vi "TestPCO.Cam.vi"() -> ()   [LabVIEW 2011]
uses:
  <vilib>/Utility/importsl/GetValueByPointer/datatype.ctl
  <vilib>/Utility/importsl/GetValueByPointer/GetValueByPointer.xnode
  National Instruments/LabVIEW 2011/resource/lvimptsl.dll
panel:
  out "End":bool
  in  "Exposure [ms]":dbl(slide) scale=1.0..100.0
  out "ActRes":cluster{"wXResAct":u16, "wYResAct":u16}
  out "Exposure [s]":dbl
  out "ImgPointer":u32
  out "sBufNr out":i16
  in  "Finish":bool
  out "Intensity Graph":u16[][](graph)
  out "bytes allocated":u32
  out "Frame":i32
  out "Handle":u64
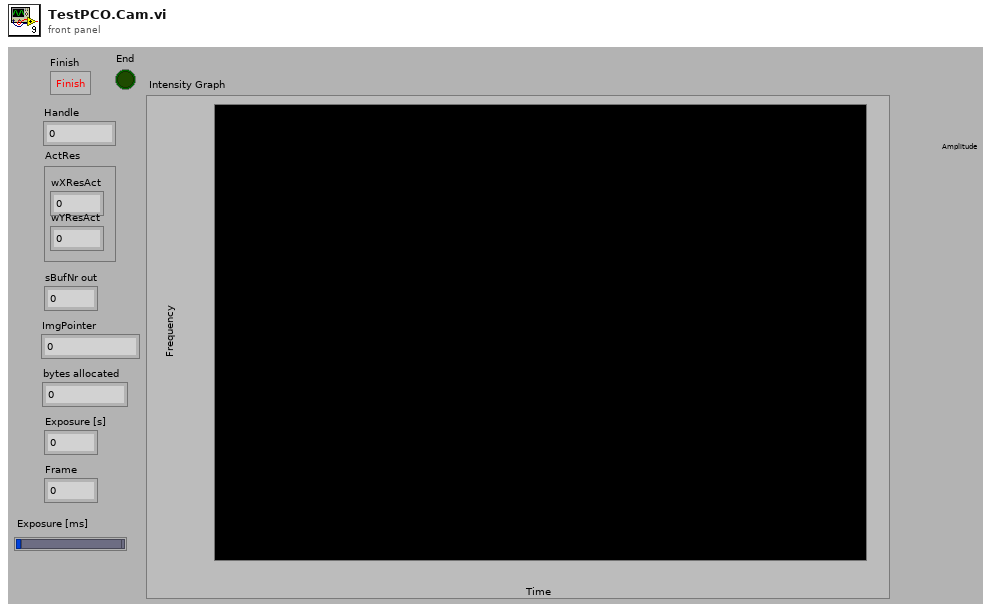
[diagram p1: front panel]
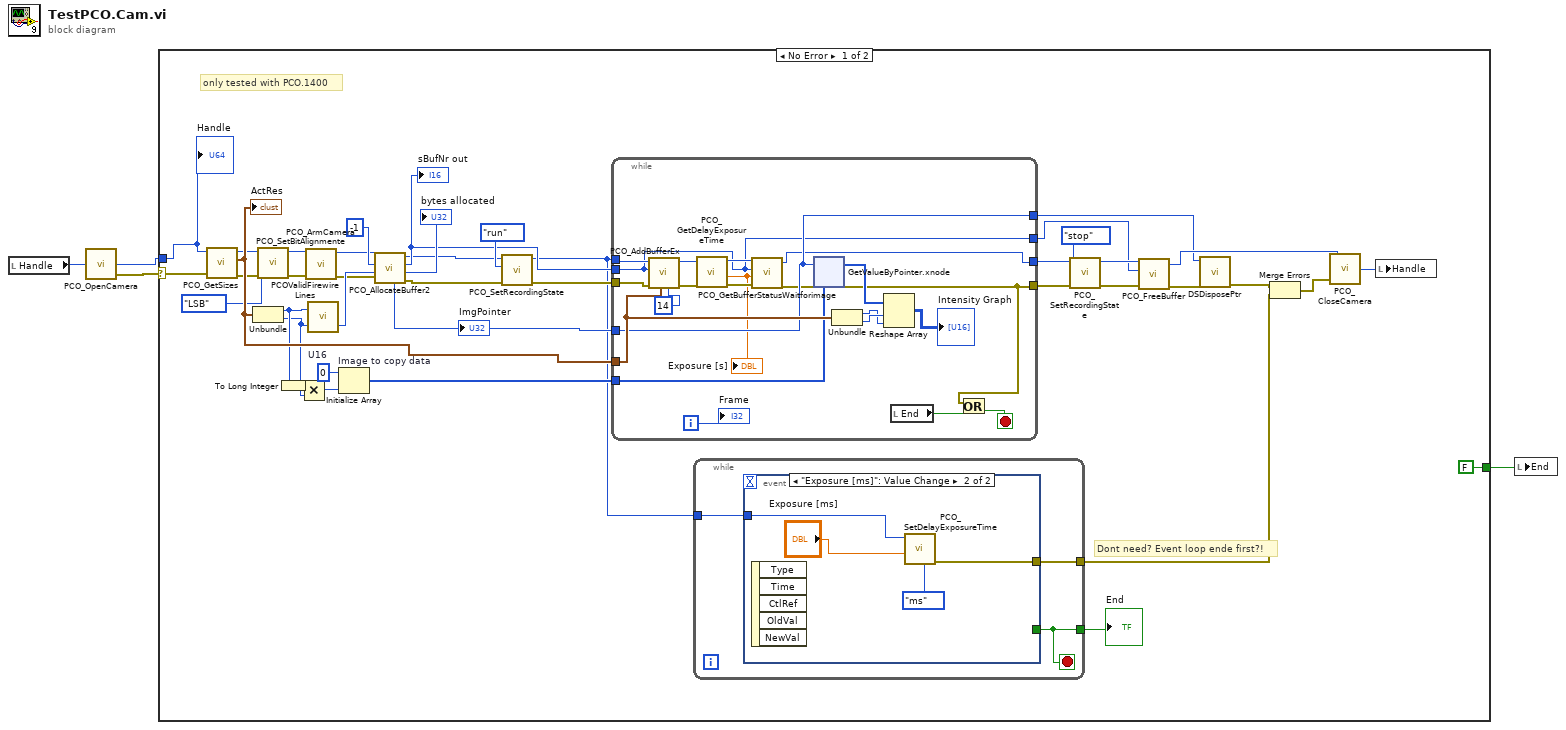
[diagram p0: block diagram]
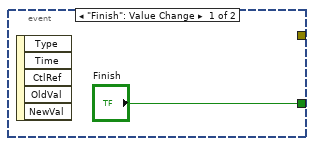
[diagram p2: hidden frame]
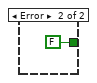
[diagram p3: hidden frame]
diagram:
  n1 = local read "Handle"() -> (w2:u64)
  n2 = call "PCO_OpenCamera.vi"("Handle (0 for new)"=w2) -> ("error out"=w4:errorcluster, "Handle Out"=w3:u64)  [unwired: 2 in, 1 out]
  n3 = case shown="No Error" w4 {
    selector: w4 -> [w34 _]
    tunnel: w3 -> [w33 _]
    tunnel: [FALSE ("End") FALSE ("End")] -> w1
    frame No Error {
      w27 = u16 0  # U16
      # "Dont need? Event loop ende first?!"
      # "only tested with PCO.1400"
      n4 = call "PCO_GetSizes.vi"("error in (no error)"=w34, "Handle"=w33) -> ("error out"=w7:errorcluster, "ActRes"=w32:cluster{"wXResAct":u16, "wYResAct":u16}, "Handle Out"=w9:u64)  [unwired: 7 out]
      "ActRes" <- w32
      n5 = Unbundle(w32) -> ("wXResAct"=w30:u16, "wYResAct"=w29:u16)
      n6 = call "PCO_SetBitAlignmente.vi"("error in (no error)"=w7, "wBitAlignment"=enum16{"MSB", "LSB"}."LSB", "Handle"=w9) -> ("error out"=w6:errorcluster, "Handle Out"=w8:u64)  [unwired: 6 in, 1 out]
      n7 = To Long Integer(number=w30) -> (32bit integer=w17:i32)
      n8 = Multiply(x=w17, y=w29) -> (x*y=w28:i32)
      n9 = call "PCO_ArmCamera.vi"("error in (no error)"=w6, "Handle"=w8) -> ("error out"=w21:errorcluster, "Handle Out"=w22:u64)  [unwired: 8 out]
      n10 = call "PCOValidFirewireLines.vi"("wYResAct"=w29, "wXResAct"=w30) -> ("ValidBytes"=w31:u32)  [unwired: 1 out]
      n11 = Initialize Array "Image to copy data"(w27, w28) -> (w26:u16[])
      n12 = call "PCO_AllocateBuffer2.vi"("error in (no error)"=w21, "PointerSize (bytes)"=w31, "sBufNr"=i16 -1, "Handle"=w22) -> ("error out"=w20:errorcluster, "bytes allocated"=→"bytes allocated":u32, "sBufNr out"=w35:i16, "Handle Out"=w19:u64, "BufferPointer"=w43:u64)  [unwired: 3 out]
      "sBufNr out" <- w35
      "ImgPointer" <- w43
      n13 = call "PCO_SetRecordingState.vi"("error in (no error)"=w20, "wRecState"=enum16{"stop", "run"}."run", "Handle"=w19) -> ("error out"=w38:errorcluster, "Handle Out"=w13:u64)  [unwired: 7 out]
      n14 = while {
        tunnel: w13 -> [w69]
        tunnel: [w60] -> w42
        tunnel: [w55] -> w41
        tunnel: w43 -> [w66]
        tunnel: w35 -> [w58]
        tunnel: w32 -> [w68]
        tunnel: w38 -> [w71]
        tunnel: w26 -> [w67]
        tunnel: [w66] -> w23
        tunnel: [w58] -> w18
        i -> [w75]
        stop <- w56 stop-if-true
        n15 = call "PCO_AddBufferEx.vi"("BitPerPixel"=u16 14, "Resolution"=w68, "error in (no error)"=w71, "sBufNr"=w58, "Handle"=w69) -> ("error out"=w64:errorcluster, "Handle Out"=w65:u64)  [unwired: 1 in, 4 out]
        n16 = call "PCO_GetDelayExposureTime.vi"("error in (no error)"=w64, "Handle"=w65) -> ("error out"=w63:errorcluster, "Exposure [s]"=w61:dbl, "Handle Out"=w62:u64)  [unwired: 7 out]
        "Exposure [s]" <- w61
        n17 = call "PCO_GetBufferStatusWaitforimage.vi"("error in"=w63, "expected seconds"=w61, "sBufNr"=w58, "Handle"=w62) -> ("error out"=w59:errorcluster, "Handle Out"=w60:u64)  [unwired: 1 out]
        n18 = xnode "GetValueByPointer.xnode"("Pointer"=w66, "InputType"=w67, "ErrorIn"=w59) -> ("Output"=w57:u16[], "ErrorOut"=w55:errorcluster)  [unwired: 1 in]
        n19 = Unbundle(w68) -> ("wXResAct"=w73:u16, "wYResAct"=w74:u16)
        n20 = Reshape Array(w57, w74, w73) -> (→"Intensity Graph":u16[][])
        n21 = local read "End"() -> (w54:bool)
        n22 = Or(x=w55, y=w54) -> (x .or. y?=w56:bool)
        "Frame" <- w75
      }
      n23 = while {
        tunnel: [w48] -> w15
        tunnel: w13 -> [w47]
        tunnel: [w46] -> w10
        stop <- w48 stop-if-true
        n24 = event shown="[1] \"Exposure [ms]\": Value Change" {
          selector: _ -> [_ _]
          dyn-events: _ -> [_ _]
          timeout: _ -> [_ _]
          tunnel: ["Finish" _] -> w48
          tunnel: w47 -> [_ w53]
          tunnel: [_ w50] -> w46
          event "Finish": Value Change {
            n25 = event-data() -> ()  [unwired: 1 in, 5 out]
          }
          event "Exposure [ms]": Value Change {
            n26 = event-data() -> ()  [unwired: 1 in, 5 out]
            n27 = call "PCO_SetDelayExposureTime.vi"("wTimebaseExposure"=enum16{"ns", "µs", "ms"}."ms", "dwExposure"="Exposure [ms]", "Handle"=w53) -> ("error out"=w50:errorcluster)  [unwired: 6 in, 2 out]
          }
        }
      }
      "End" <- w15
      n28 = call "PCO_SetRecordingState.vi"("error in (no error)"=w41, "wRecState"=enum16{"stop", "run"}."stop", "Handle"=w42) -> ("error out"=w37:errorcluster, "Handle Out"=w36:u64)  [unwired: 7 out]
      n29 = call "PCO_FreeBuffer.vi"("error in (no error)"=w37, "sBufNr"=w18, "Handle"=w36) -> ("error out"=w24:errorcluster, "Handle Out"=w25:u64)  [unwired: 7 out]
      n30 = call <vilib>:"DSDisposePtr.vi"("error in (no error)"=w24, "Pointer"=w23) -> ("error out"=w12:errorcluster)  [unwired: 9 in]
      n31 = Merge Errors(w12, w10) -> (w11:errorcluster)
      n32 = call "PCO_CloseCamera.vi"("error in (no error)"=w11, "Handle"=w25) -> ("Handle Out (success:0, otherwise input)"=w16:u32)  [unwired: 1 in, 2 out]
      n33 = local write "Handle"(w16) -> ()
      "Handle" <- w33
    }
    frame Error {
    }
  }
  n34 = local write "End"(w1) -> ()
